vi "getTemperature.vi"() -> (0 "error out":errorcluster, 3 "Measured Temperature [*C]":dbl)   [LabVIEW 2015]
uses:
  <vilib>/myRIO/Instrument Drivers/Onboard IO/I2C/vis/Configure.vi
  <vilib>/myRIO/Instrument Drivers/Onboard IO/I2C/vis/Write.vi
  <vilib>/myRIO/Instrument Drivers/Onboard IO/I2C/vis/Read.vi
  <vilib>/myRIO/Instrument Drivers/Onboard IO/I2C/vis/Smart Open.vi
  <vilib>/Utility/error.llb/Error Cluster From Error Code.vi
  <vilib>/myRIO/Common/Instrument Driver Framework/myRIO v1.0/I2C/vis/myRIO v1.0 Configure I2C.vi
  <vilib>/myRIO/Common/Instrument Driver Framework/myRIO v1.0/I2C/vis/myRIO v1.0 Write I2C.vi
  <vilib>/myRIO/Common/Instrument Driver Framework/myRIO v1.0/I2C/vis/myRIO v1.0 Read I2C.vi
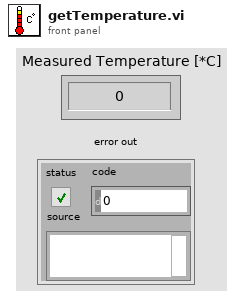
[diagram p1: front panel]
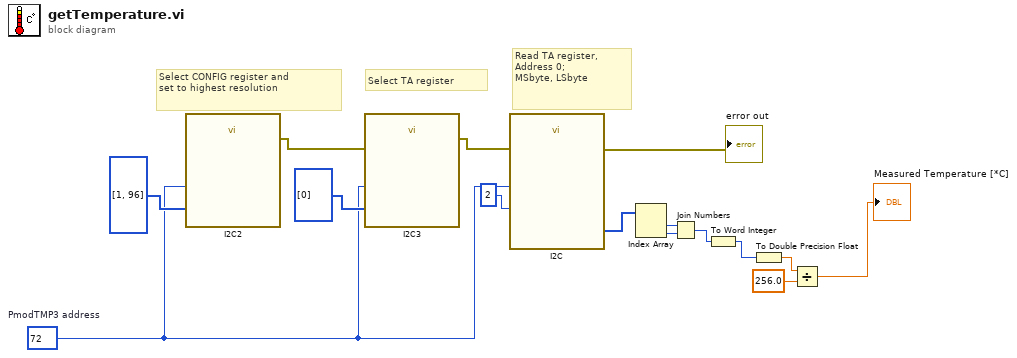
[diagram p0: block diagram]
diagram:
  w5 = u8 72  # PmodTMP3 address
  # "Select TA register"
  # "Select CONFIG register and\nset to highest resolution"
  # "Read TA register,\nAddress 0;\nMSbyte, LSbyte"
  n1 = call "I2C2"("Slave Address (7-bit)"=w5, "Bytes to Write"=u8[] [1, 96]) -> ("error out"=w4:errorcluster)  [unwired: 25 in]
  n2 = call "I2C3"("Slave Address (7-bit)"=w5, "Bytes to Write"=u8[] [0], "error in (no error)"=w4) -> ("error out"=w3:errorcluster)  [unwired: 24 in]
  n3 = call "I2C"("Slave Address (7-bit)"=w5, "Byte Count"=u32 2, "error in (no error)"=w3) -> ("Bytes Read"=w9:u8[], "error out"=→"error out":errorcluster)  [unwired: 23 in]
  n4 = Index Array "Index Array"(array=w9) -> (element #1=w13:u8, element #2=w12:u8)  [unwired: 2 in]
  n5 = Join Numbers(hi=w13, lo=w12) -> ((hi.lo)=w11:u16)
  n6 = To Word Integer(number=w11) -> (16bit integer=w10:i16)
  n7 = To Double Precision Float(number=w10) -> (double precision float=w15:dbl)
  n8 = Divide(x=w15, y=256.0) -> (x/y=→"Measured Temperature [*C]":dbl)
